vi "Update.vi"(8 "error in":errorcluster, 10 "Update":T1, 11 "SplashScreen in":T2) -> (0 "error out":errorcluster, 3 "SplashScreen out":T2)   [LabVIEW 2013, in "RT Temperature Controller.lvlib" / "splash screen.lvlib"]
uses:
  splash screen.lvlib
  splash screen.ctl
  notifier data.ctl
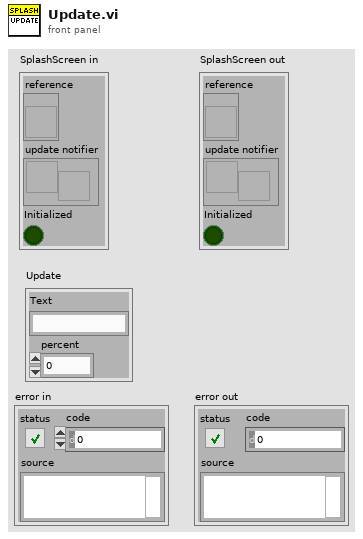
[diagram p1: front panel]
types:
  T1 = typedef "RT Temperature Controller.lvlib/splash screen.lvlib/notifier data.ctl" = cluster{"Text":string, "percent":dbl}
  T2 = typedef "RT Temperature Controller.lvlib/splash screen.lvlib/splash screen.ctl" = cluster{"reference":refnum<vi>, "update notifier":refnum<notifier>, "Initialized":bool}
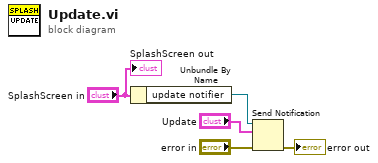
[diagram p0: block diagram]
diagram:
  n1 = Unbundle By Name("SplashScreen in") -> ("update notifier"=w5:refnum<notifier>)
  n2 = Send Notification(notification="Update", notifier=w5, error in (no error)="error in") -> (error out=→"error out":errorcluster)  [unwired: 1 out]
  "SplashScreen out" <- "SplashScreen in"
